vi "Normalize Waveform.vi"(8 "error in (no error)":errorcluster, 11 "waveform in":waveform(dbl)) -> (0 "error out":errorcluster, 1 "offset":dbl format="%0.2f", 2 "scale":dbl format="%0.2f", 3 "normalized waveform":waveform(dbl))   [LabVIEW 2011]
doc: "Determines the <B>scale</B> and <B>offset</B> necessary to transform the waveform data so that its maximum is 1.00 and its minimum is -1.00."
uses:
  NI_AALBase.lvlib
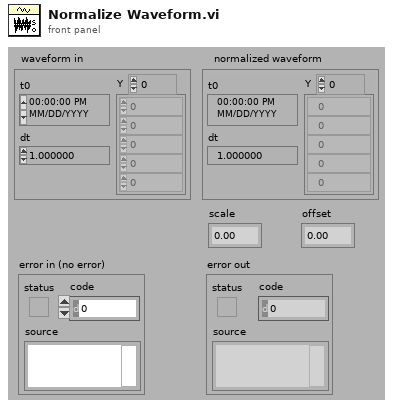
[diagram p1: front panel]
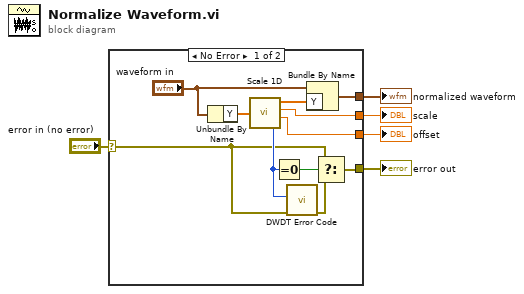
[diagram p0: block diagram]
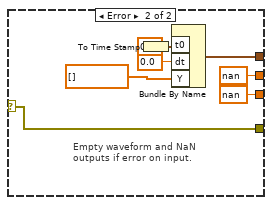
[diagram p2: hidden frame]
diagram:
  n1 = case shown="No Error" "error in (no error)" {
    selector: "error in (no error)" -> [w7 w24]
    tunnel: [w15 w21] -> w5
    tunnel: [w14 nan ("offset")] -> w4
    tunnel: [w13 nan ("scale")] -> w3
    tunnel: [w9 w24] -> w2
    frame No Error {
      n2 = Unbundle By Name("waveform in") -> ("Y"=w11:dbl[])
      n3 = call "Scale 1D.vi"("X"=w11) -> ("Y=(X-offset)/scale"=w12:dbl[], "scale"=w13:dbl, "offset"=w14:dbl, "error"=w8:i32)
      n4 = Equal To 0?(x=w8) -> (x = 0?=w10:bool)
      n5 = call "DWDT Error Code.vi"("error in (no error)"=w7, "error code"=w8) -> ("error out"=w6:errorcluster)  [unwired: 9 out]
      n6 = Bundle By Name(cluster="waveform in", "Y"=w12) -> (w15:waveform(dbl))
      n7 = Select(t=w7, s=w10, f=w6) -> (s? t:f=w9:errorcluster)
    }
    frame Error {
      # "Empty waveform and NaN\noutputs if error on input."
      n8 = To Time Stamp(1:0.0 ("t0")) -> (0:w17:timestamp)
      n9 = Bundle By Name("t0"=w17, "dt"=0.0, "Y"=dbl[] []) -> (w21:waveform(dbl))  [unwired: 1 out]
    }
  }
  "normalized waveform" <- w5
  "scale" <- w3
  "offset" <- w4
  "error out" <- w2
